vi "Render.vi"(8 "error in (no error)":errorcluster, 10 "String in":string, 11 "Blockquote in":refnum<class "Blockquote.lvclass">) -> (0 "error out":errorcluster, 2 "String out":string, 3 "Blockquote out":refnum<class "Blockquote.lvclass">)   [LabVIEW 2021, in "LvMarkdown.lvlib" / "Blockquote.lvclass"]
uses:
  Blockquote.lvclass
  C:/GitHub/LvMarkdown/src/LvMarkdown/Markdown.lvclass
  GetBlockquoteTag.vi
  Blockquote.lvclass/Blockquote.ctl
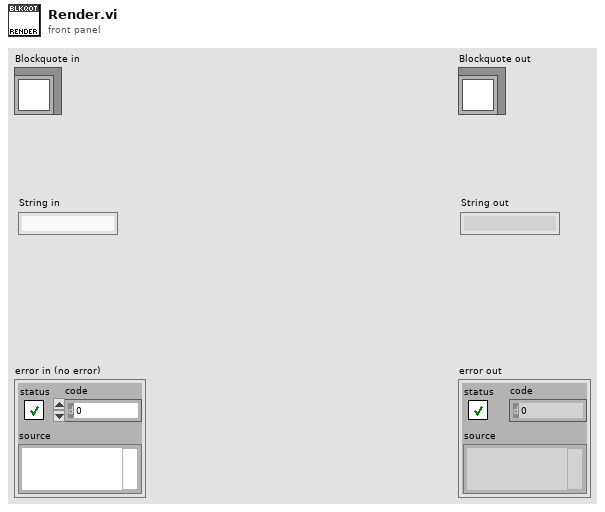
[diagram p1: front panel]
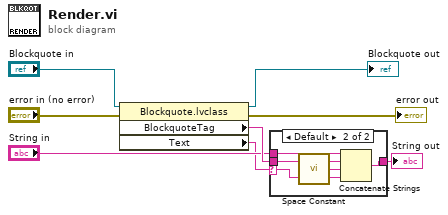
[diagram p0: block diagram]
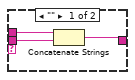
[diagram p2: hidden frame]
diagram:
  n1 = property class="Blockquote.lvclass"(reference="Blockquote in", error in="error in (no error)") -> (reference out=→"Blockquote out":refnum<class "Blockquote.lvclass">, error out=→"error out":errorcluster, "BlockquoteTag"=w6:string, "Text"=w3:string)
  n2 = case shown="Default" w3 {
    selector: w3 -> [_ w13]
    tunnel: w6 -> [w10 w16]
    tunnel: "String in" -> [w11 w15]
    tunnel: [w9 w14] -> w4
    frame "" {
      n3 = Concatenate Strings(w11, w10) -> (w9:string)
    }
    frame Default {
      n4 = call <vilib>:"Space Constant.vi"() -> ("String"=w12:string)
      n5 = Concatenate Strings(w15, w16, w12, w13) -> (w14:string)
    }
  }
  "String out" <- w4
